vi "Read Motors.vi"(8 "error in (no error)":errorcluster, 11 "Fuji Delta Robot in":refnum<class "Fuji Delta Robot.lvclass">) -> (0 "error out":errorcluster, 2 "Motors":refnum<class "FujiMotor.lvclass">[](array[class]), 3 "Fuji Delta Robot out":refnum<class "Fuji Delta Robot.lvclass">)   [LabVIEW 2014, in "Fuji Delta Robot.lvlib" / "Fuji Delta Robot.lvclass"]
uses:
  Fuji Delta Robot.lvclass
  ALPHA5 RS485/Classes/FujiMotor/FujiMotor.lvclass
  Fuji Delta Robot.lvclass/Fuji Delta Robot.ctl
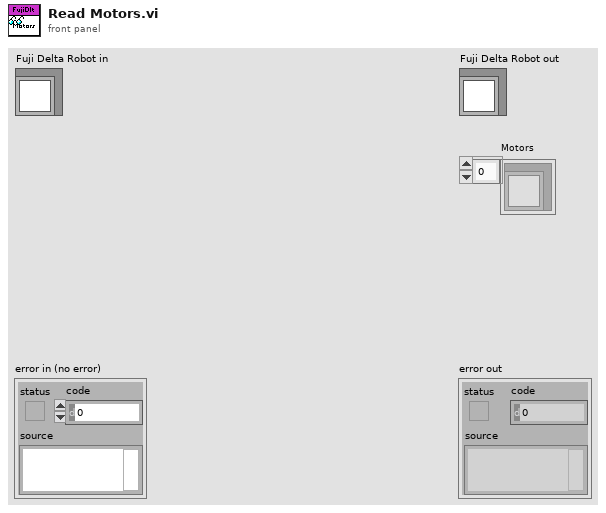
[diagram p1: front panel]
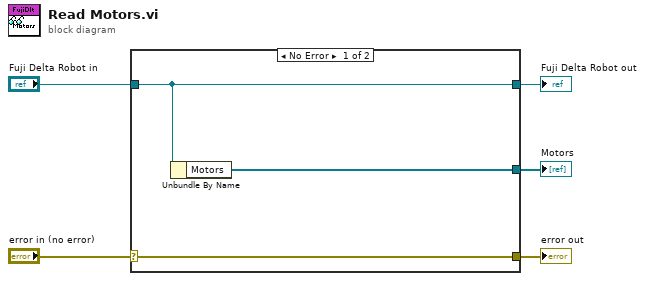
[diagram p0: block diagram]
diagram:
  n1 = case shown="No Error" "error in (no error)" {
    selector: "error in (no error)" -> [w8 w9]
    tunnel: [w8 w9] -> w4
    tunnel: [w7 w10] -> w2
    tunnel: "Fuji Delta Robot in" -> [w7 w10]
    tunnel: [w6 _] -> w1
    frame No Error {
      n2 = Unbundle By Name(w7) -> ("Motors"=w6:refnum<class "FujiMotor.lvclass">[])
    }
    frame Error {
    }
  }
  "error out" <- w4
  "Fuji Delta Robot out" <- w2
  "Motors" <- w1
